vi "Send Write Control cluster.vi"(7 "Message Priority (Normal)":T2=enum."Normal", 8 "error in (no error)":errorcluster, 10 "Control cluster":T1={"Number of points"=816000.0, "Input Range"=10000, "Trigger Level"=29, "Trigger source"=TRUE} {"Trigger Level" min=-100 max=100 step=1 scale=-100.0..100.0; "Input Range" items=["+/- 5 V"=10000, "+/- 2 V"=4000, "+/- 1 V"=2000, "+/- 500 mV"=1000, "+/- 200 mV"=400, "+/- 100 mV"=200]; "Number of points" min=160.0 step=160.0}, 11 "Message Enqueuer":refnum<class "Message Enqueuer.lvclass">) -> (0 "error out":errorcluster, 3 "Message Enqueuer out":refnum<class "Message Enqueuer.lvclass">)   [LabVIEW 2015, in "Write Control cluster Msg.lvclass"]
doc: "This VI sends the message to an actor."
uses:
  Write Control cluster Msg.lvclass
  <vilib>/ActorFramework/Message Enqueuer/Message Enqueuer.lvclass
  <vilib>/ActorFramework/Message Enqueuer/Message Priority.ctl
  Basic controlls.ctl
  Write Control cluster Msg.lvclass/Write Control cluster Msg.ctl
  <vilib>/ActorFramework/Message Enqueuer/Message Enqueuer.lvclass/Message Enqueuer.ctl
  <vilib>/ActorFramework/Message Priority Queue/Priority Enqueue.vi
panel:
  # "Basic Card Controlls"
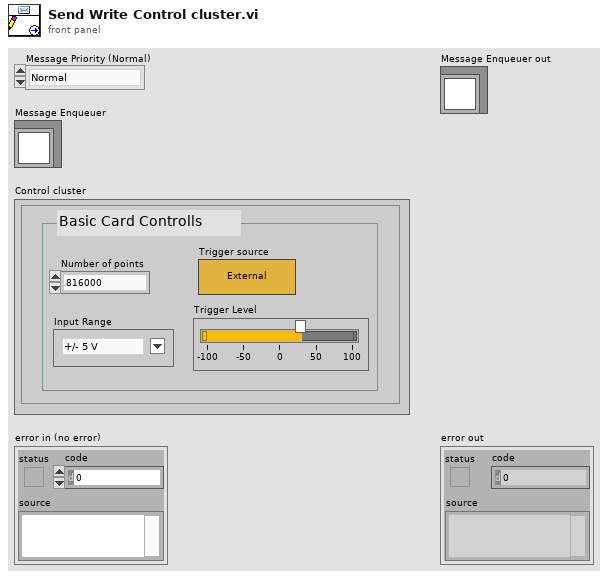
[diagram p1: front panel]
types:
  T1 = typedef "Basic controlls.ctl" = cluster{"Number of points":dbl, "Input Range":u32, "Trigger Level":i32, "Trigger source":bool}
  T2 = typedef "Actor Framework.lvlib/Message Enqueuer.lvclass/Message Priority.ctl" = enum16{"Low", "Normal", "High"}
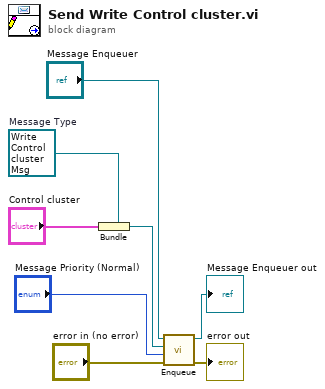
[diagram p0: block diagram]
diagram:
  w5 = refnum<class "Write Control cluster Msg.lvclass"> refnum  # Message Type
  n1 = Bundle(cluster=w5, "Control cluster") -> (w4:refnum<class "Write Control cluster Msg.lvclass">)
  n2 = call <vilib>:"Enqueue.vi"("error in (no error)"="error in (no error)", "Message Priority (Normal)"="Message Priority (Normal)", "Message"=w4, "Message Enqueuer in"="Message Enqueuer") -> ("error out"=→"error out":errorcluster, "Message Enqueuer out"=→"Message Enqueuer out":refnum<class "Message Enqueuer.lvclass">)  [unwired: 6 in]
